vi "Review Intermediate Result.vi"(0 "Vector Path in":refnum<class "Vector Abstract Path.lvclass">, 5 "One-Port Charact Data In":T1, 11 "error in (no error)":errorcluster) -> (4 "Vector Path out":refnum<class "Vector Abstract Path.lvclass">, 6 "Response":string, 8 "One-Port Charact Data Out":T1, 15 "error out":errorcluster)   [LabVIEW 2023, in "RFFixtureCharact.Public.lvlib" / "Vector Abstract Path.lvclass"]
uses:
  Vector Abstract Path.lvclass
  Instruments/Cal Standard/Type Definitions/One-Port Charact Data.ctl
  Instruments/Cal Standard/Type Definitions/Standard Type.ctl
  Vector Abstract Path.lvclass/Vector Abstract Path.ctl
  Instruments/RFFixtureCharact.Instruments.lvlib
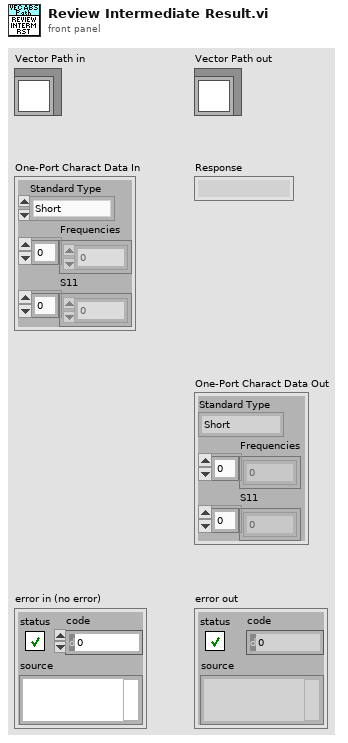
[diagram p1: front panel]
types:
  T1 = typedef "RFFixtureCharact.Instruments.lvlib/One-Port Charact Data.ctl" = cluster{"Standard Type":T2, "Frequencies":dbl[], "S11":cdb[]}
  T2 = typedef "RFFixtureCharact.Instruments.lvlib/Standard Type.ctl" = enum16{"Short", "Open", "Load", "PowerMeter", "None"}
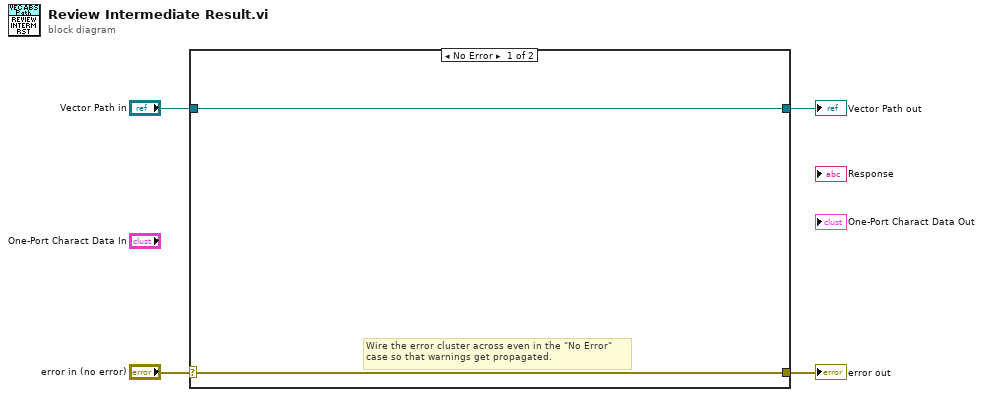
[diagram p0: block diagram]
diagram:
  n1 = case shown="No Error" "error in (no error)" {
    selector: "error in (no error)" -> [w5 w8]
    tunnel: [w5 w8] -> w3
    tunnel: [w6 w7] -> w1
    tunnel: "Vector Path in" -> [w6 w7]
    frame No Error {
      # "Wire the error cluster across even in the \"No Error\"\ncase so that warnings get propagated."
    }
    frame Error {
    }
  }
  "error out" <- w3
  "Vector Path out" <- w1
